vi "Check All Stopped.vi"(8 "error in (no error)":errorcluster, 11 "Log Manager Module in":refnum<class "Log Manager Module.lvclass">) -> (0 "error out":errorcluster, 2 "All Idle":bool, 3 "Log Manager Module out":refnum<class "Log Manager Module.lvclass">)   [LabVIEW 2020, in "VolatusData.lvlib" / "Log Manager Module.lvclass"]
uses:
  Log Manager Module.lvclass
  C:/dev/lv20CE/relink/lv-volatus/Volatus/Module/Module.lvclass
  Log Manager Module.lvclass/Log Manager Module.ctl
  Logger State.ctl
  Logging State.ctl
  Volatus/Module/Module.lvclass/Module.ctl
  Volatus/Module/Module.lvclass
  VolatusData.lvlib
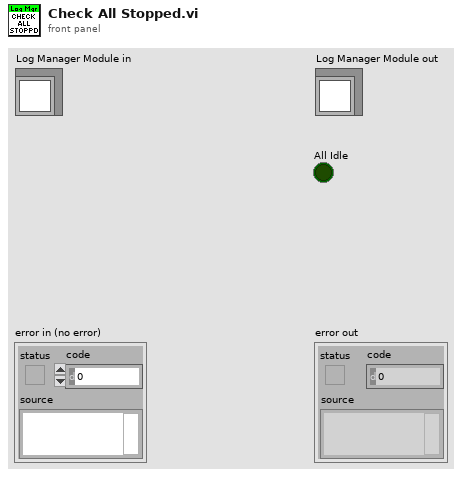
[diagram p1: front panel]
types:
  T1 = typedef "VolatusData.lvlib/Log Manager Module.lvclass/Logger.ctl" = cluster{"ID":string, "MsgQ":refnum<class "MessageQ.lvclass">, "State":T2}
  T2 = typedef "VolatusData.lvlib/Logger State.ctl" = enum16{"Unknown", "Idle", "Preparing", "Ready", "Logging", "Stopping"}
  T3 = typedef "VolatusData.lvlib/Logging State.ctl" = enum16{"Idle", "Starting", "Logging", "Stopping"}
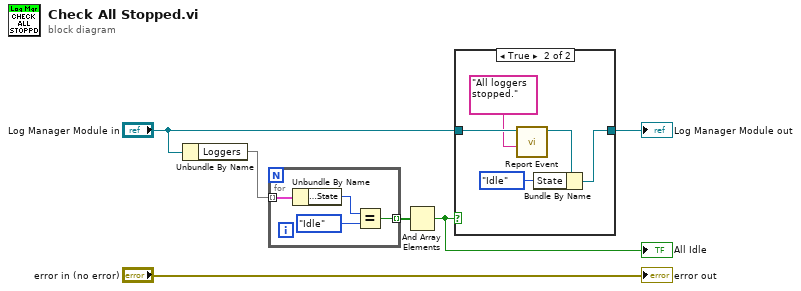
[diagram p0: block diagram]
diagram:
  n1 = Unbundle By Name("Log Manager Module in") -> ("Loggers"=w3:map{string, T1})
  n2 = for {
    tunnel: w3 -> [w10] mode=indexing
    tunnel: [w7] -> w5 mode=indexing
    n3 = Unbundle By Name(w10) -> ("Logger.State"=w9:T2)
    n4 = Equal?(x=w9, y=Logger_State."Idle") -> (x = y?=w7:bool)
  }
  n5 = And Array Elements(Boolean array=w5) -> (logical AND=w4:bool)
  "All Idle" <- w4
  n6 = case shown="True" w4 {
    tunnel: "Log Manager Module in" -> [w11 w16]
    tunnel: [w11 w12] -> w1
    frame False {
    }
    frame True {
      n7 = call "Report Event.vi"("Message"="All loggers stopped.", "Module in"=w16) -> ("Module out"=w14:refnum<class "Log Manager Module.lvclass">)  [unwired: 8 in, 1 out]
      n8 = Bundle By Name(cluster=w14, "State"=Logging_State."Idle") -> (w12:refnum<class "Log Manager Module.lvclass">)
    }
  }
  "Log Manager Module out" <- w1
  "error out" <- "error in (no error)"
